vi "ReverseEncoderDirection.vi"(8 "error in":errorcluster, 10 "Axis":enum16{"Z", "Y", "X"}(ring), 11 "connection refnum in":refnum<k5>) -> (0 "error out":errorcluster, 2 "Reverse/Normal?":string, 3 "connection refnum out":refnum<k5>)   [LabVIEW 2023]
uses:
  GlobalVarsNetwork.vi
panel:
  out "New":bool[](array[boolean])
  out "Original":bool[](array[boolean])
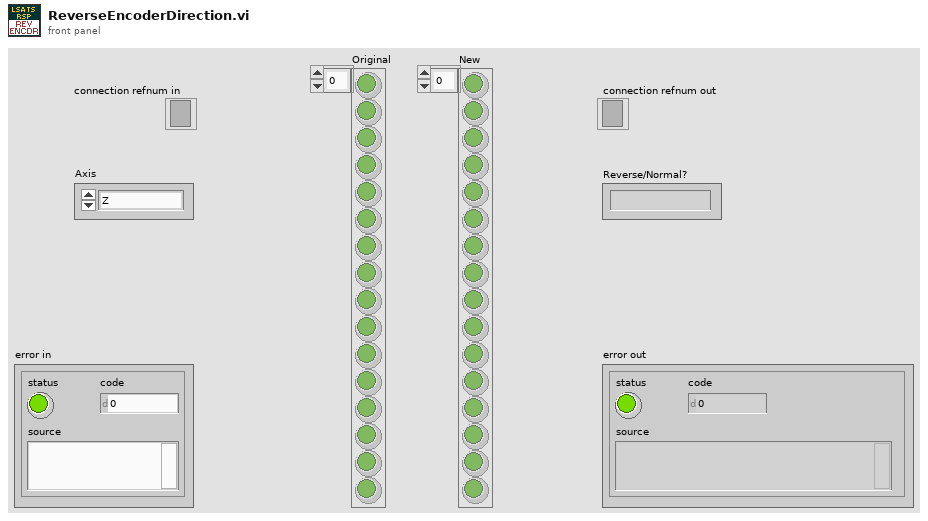
[diagram p1: front panel]
types:
  T1 = cluster{"XY_IP_ADDRESS":string, "Z_IP_ADDRESS":string, "Port":u16, "connection refnum x,y":refnum<k5>, "connection refnum z":refnum<k5>}
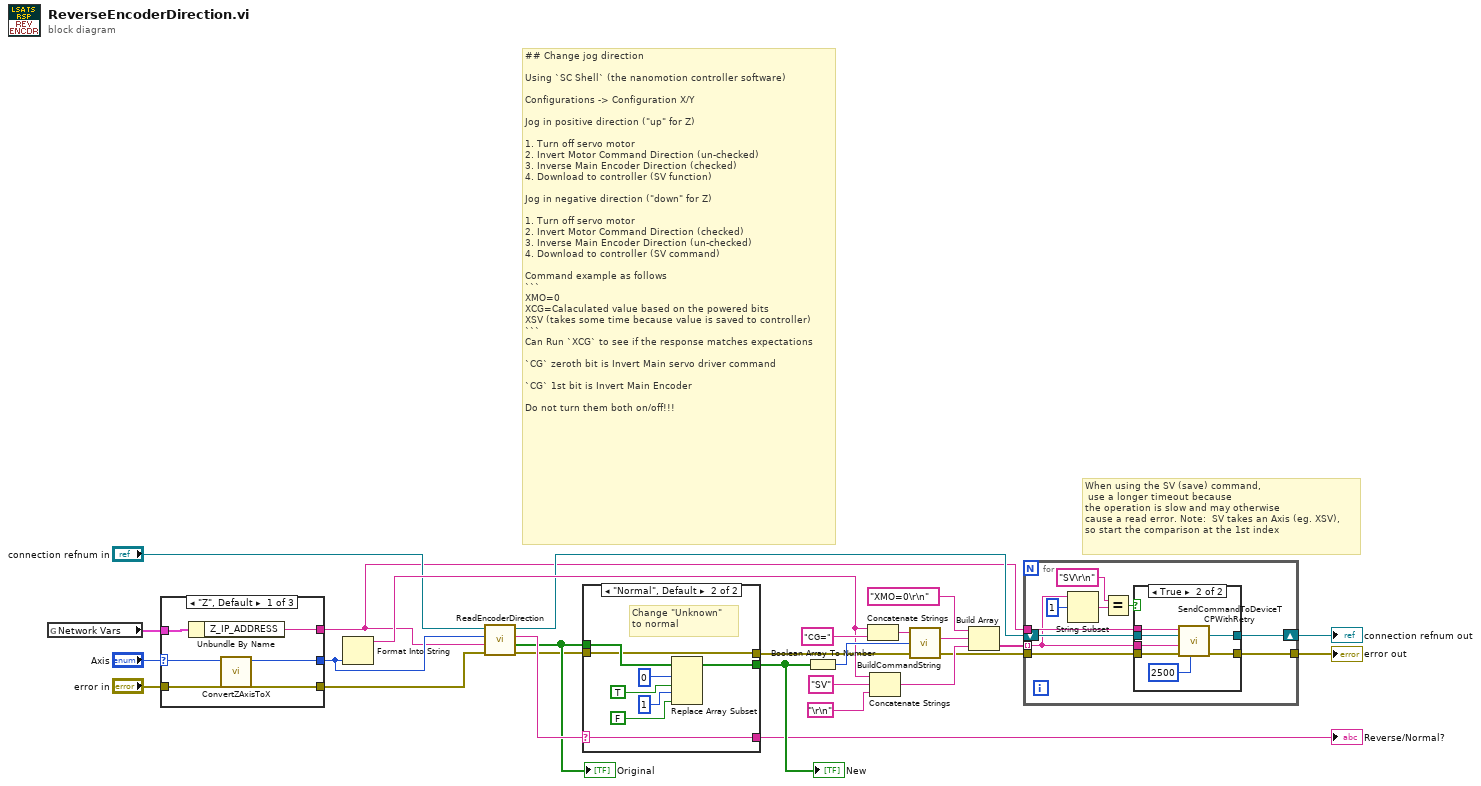
[diagram p0: block diagram]
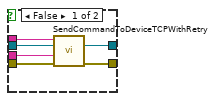
[diagram p2: hidden frame]
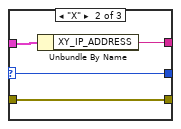
[diagram p3: hidden frame]
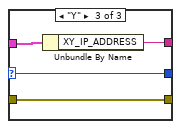
[diagram p4: hidden frame]
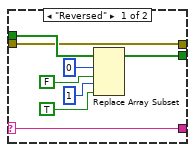
[diagram p5: hidden frame]
diagram:
  # "When using the SV (save) command,\n use a longer timeout because \nthe operation is slow and may otherwise\ncause a read error. Note:  SV takes an Axis (eg. XSV), \nso start the comparison at the 1st index"
  # "## Change jog direction\n\nUsing `SC Shell` (the nanomotion controller software)\n\nConfigurations -> Configuration X/Y\n\nJog in positive direction (\"up\" for Z)\n\n1. Turn off servo motor\n2. Invert Motor Command Direction (un-checked)\n3. Inverse Main Encoder Direction (checked)\n4. Download to controller (SV function)\n\nJog in negative direction (\"down\" for Z)\n\n1. Turn off servo motor\n2. Invert Motor Command Direction (checked)\n3. Inverse Main Encoder Direction (un-checked)\n4. Download to controller (SV command)\n\nCommand example as follows\n```\nXMO=0\nXCG=Calaculated value based on the powered bits\nXSV (takes some time because value is saved to controller)\n```\nCan Run `XCG` to see if the response matches expectations\n\n`CG` zeroth bit is Invert Main servo driver command\n\n`CG` 1st bit is Invert Main Encoder\n\nDo not turn them both on/off!!!"
  n1 = global read "GlobalVarsNetwork.vi" "Network Vars"() -> (w25:T1)
  n2 = case shown="\"Z\", Default" "Axis" {
    selector: "Axis" -> [w31 w34 w38]
    tunnel: w25 -> [w32 w36 w40]
    tunnel: [w30 w34 w38] -> w6
    tunnel: [w29 w35 w39] -> w1
    tunnel: "error in" -> [w28 w33 w37]
    tunnel: [w28 w33 w37] -> w8
    frame "Z", Default {
      n3 = Unbundle By Name(w32) -> ("Z_IP_ADDRESS"=w29:string)
      n4 = call "ConvertZAxisToX.vi"("Axis in"=w31) -> ("Axis out"=w30:enum16{"Z", "Y", "X"})  [unwired: 6 in]
    }
    frame "X" {
      n5 = Unbundle By Name(w36) -> ("XY_IP_ADDRESS"=w35:string)
    }
    frame "Y" {
      n6 = Unbundle By Name(w40) -> ("XY_IP_ADDRESS"=w39:string)
    }
  }
  n7 = Format Into String(w6) -> (resulting string=w18:string)  [unwired: 3 in, 1 out]
  n8 = call "ReadEncoderDirection.vi"("error in"=w8, "IP address"=w1, "Axis"=w6, "connection refnum in"="connection refnum in") -> ("error out"=w4:errorcluster, "Boolean Array"=w5:bool[], "Encoder Direction"=w7:string, "connection refnum out"=w9:refnum<k5>)  [unwired: 4 in]
  "Original" <- w5
  n9 = case shown="\"Normal\", Default" w7 {
    selector: w7 -> [w42 w50]
    tunnel: w5 -> [w44 w54]
    tunnel: [w43 w53] -> w27
    tunnel: [w42 w50] -> w2
    tunnel: w4 -> [w41 w49]
    tunnel: [w41 w49] -> w3
    frame "Reversed" {
      n10 = Replace Array Subset(array=w44, new element #1=FALSE, index #1=0 ("index"), new element #2=TRUE, index #2=1 ("index")) -> (w43:bool[])
    }
    frame "Normal", Default {
      # "Change \"Unknown\"\nto normal"
      n11 = Replace Array Subset(array=w54, new element #1=TRUE, index #1=0 ("index"), new element #2=FALSE, index #2=1 ("index")) -> (w53:bool[])
    }
  }
  "New" <- w27
  "Reverse/Normal?" <- w2
  n12 = Boolean Array To Number(Boolean array=w27) -> (number=w24:u32)
  n13 = Concatenate Strings(w18, "CG=" ("string")) -> (w22:string)
  n14 = Concatenate Strings(w18, "SV" ("string"), "\r\n") -> (w16:string)
  n15 = call "BuildCommandString.vi"("error in"=w3, "Numeric Value"=w24, "Command"=w22) -> ("error out"=w15:errorcluster, "Result"=w20:string)  [unwired: 1 in]
  n16 = Build Array("XMO=0\r\n" ("string"), w20, w16) -> (w21:string[])
  n17 = for {
    tunnel: w1 -> [w66]
    tunnel: w21 -> [w60] mode=indexing
    tunnel: w15 -> [w65]
    tunnel: [w64] -> w13
    shift-right: [w63] -> w12
    shift-left: w9 -> [w62]
    n18 = String Subset(string=w60, offset (0)=1) -> (substring=w58:string)  [unwired: 1 in]
    n19 = Equal?(x="SV\r\n", y=w58) -> (x = y?=w61:bool)
    n20 = case shown="True" w61 {
      tunnel: w66 -> [w72 w79]
      tunnel: w65 -> [w67 w74]
      tunnel: [w71 w73] -> w64
      tunnel: w60 -> [w70 w76]
      tunnel: [w69 w77] -> w63
      tunnel: w62 -> [w68 w78]
      frame False {
        n21 = call "SendCommandToDeviceTCPWithRetry.vi"("error in"=w67, "str command"=w70, "connection refnum in"=w68, "IP address"=w72) -> ("error out"=w71:errorcluster, "connection refnum out"=w69:refnum<k5>)  [unwired: 4 in, 2 out]
      }
      frame True {
        n22 = call "SendCommandToDeviceTCPWithRetry.vi"("timeout ms"=2500, "error in"=w74, "str command"=w76, "connection refnum in"=w78, "IP address"=w79) -> ("error out"=w73:errorcluster, "connection refnum out"=w77:refnum<k5>)  [unwired: 3 in, 2 out]
      }
    }
  }
  "error out" <- w13
  "connection refnum out" <- w12
